vi "LPC set wavelength.vi"(8 "error in (no error)":errorcluster, 10 "wavelength":dbl[unit]=8.300000000000001e-07, 11 "VISA resource name":refnum<visa-resource-name>="GPIB0::8::INSTR") -> (0 "error out":errorcluster, 3 "VISA resource name out":refnum<visa-resource-name>)   [LabVIEW 2009, in "Laser Power Controller.lvclass"]
doc: "Sets the wavelength of the LPC (laser power controller)."
uses:
  Laser Power Controller.lvclass
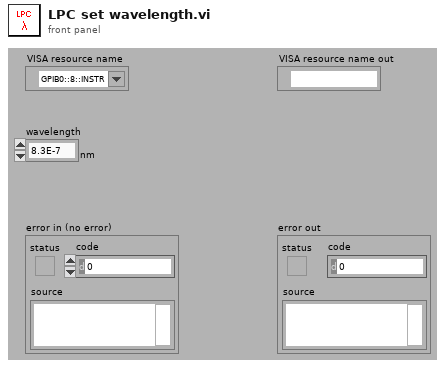
[diagram p1: front panel]
types:
  T1 = typedef "Semaphore RefNum" = refnum<k1>
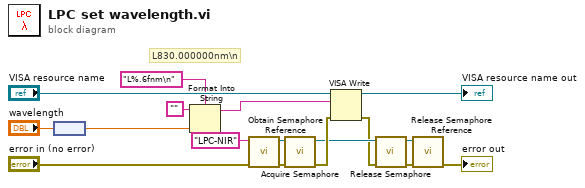
[diagram p0: block diagram]
diagram:
  # "L830.000000nm\\n"
  n1 = node("wavelength") -> (w11:dbl)
  n2 = Format Into String(format string="L%.6fnm\n", initial string="", w11) -> (resulting string=w9:string)  [unwired: 1 in, 1 out]
  n3 = call <vilib>:"Obtain Semaphore Reference.vi"("error in (no error)"="error in (no error)", "name (unnamed)"="LPC-NIR") -> ("error out"=w8:errorcluster, "semaphore"=w7:T1)  [unwired: 1 in, 3 out]
  n4 = call <vilib>:"Acquire Semaphore.vi"("error in (no error)"=w8, "semaphore"=w7) -> ("error out"=w4:errorcluster, "semaphore out"=w3:T1)  [unwired: 1 in, 3 out]
  n5 = VISA Write(VISA resource name="VISA resource name", write buffer=w9, error in (no error)=w4) -> (VISA resource name out=→"VISA resource name out":refnum<visa-resource-name>, error out=w2:errorcluster)  [unwired: 1 out]
  n6 = call <vilib>:"Release Semaphore.vi"("error in (no error)"=w2, "semaphore"=w3) -> ("error out"=w6:errorcluster, "semaphore out"=w5:T1)  [unwired: 4 out]
  n7 = call <vilib>:"Release Semaphore Reference.vi"("error in (no error)"=w6, "semaphore"=w5) -> ("error out"=→"error out":errorcluster)  [unwired: 9 out]
